vi "PRAMMS-READSTR.vi"(0 "String":string) -> (1 "Signature":u32, 2 "Length":u32, 3 "Type":u32)   [LabVIEW 2011]
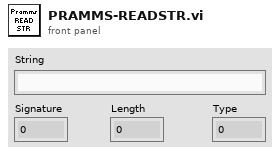
[diagram p1: front panel]
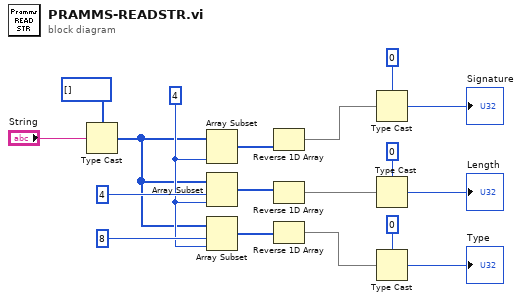
[diagram p0: block diagram]
diagram:
  w16 = 4 ("length")
  n1 = Type Cast(type=u8[] [], x="String") -> (*(type *) &x=w7:u8[])
  n2 = Array Subset(array=w7, length=w16) -> (w6:u8[])  [unwired: 1 in]
  n3 = Array Subset(array=w7, index=4, length=w16) -> (w2:u8[])
  n4 = Array Subset(array=w7, index=8, length=w16) -> (w4:u8[])
  n5 = Reverse 1D Array(array=w6) -> (reversed array=w5:u8[])
  n6 = Reverse 1D Array(array=w2) -> (reversed array=w1:u8[])
  n7 = Reverse 1D Array(array=w4) -> (reversed array=w3:u8[])
  n8 = Type Cast(type=u32 0, x=w5) -> (*(type *) &x=→"Signature":u32)
  n9 = Type Cast(type=u32 0, x=w1) -> (*(type *) &x=→"Length":u32)
  n10 = Type Cast(type=u32 0, x=w3) -> (*(type *) &x=→"Type":u32)
